vi "get data definition.vi"(10 "channel classification":T1, 11 "AppStateMachine runtime in":refnum<class "AppStateMachine runtime.lvclass">) -> (1 "valid?":bool, 2 "index cluster":variant, 3 "AppStateMachine runtime out":refnum<class "AppStateMachine runtime.lvclass">)   [LabVIEW 2017, in "AppStateMachine runtime.lvclass"]
uses:
  AppStateMachine runtime.lvclass
  <vilib>/NI/Tag Bus Module Framework/channel/channel classification.ctl
  input user data.ctl
  output user data.ctl
  parameter user data.ctl
  result user data.ctl
  <vilib>/NI/Tag Bus Module Framework/channel/TBM channel.lvclass
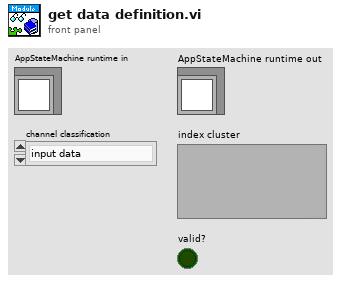
[diagram p1: front panel]
types:
  T1 = typedef "TBM channel.lvclass/channel classification.ctl" = enum16{"input data", "output data", "processing parameter", "processing result"}
  T2 = typedef "AppStateMachine runtime.lvclass/input user data.ctl" = cluster{"fmwk_placeholder":i32}
  T3 = typedef "AppStateMachine runtime.lvclass/output user data.ctl" = cluster{"fmwk_placeholder":i32}
  T4 = typedef "AppStateMachine runtime.lvclass/parameter user data.ctl" = cluster{"CPU":dbl, "Memory":dbl, "Disk":dbl}
  T5 = typedef "AppStateMachine runtime.lvclass/result user data.ctl" = cluster{"State":u16, "LED_Enable":bool, "LED_BlinksPerCycle":i32, "LED_GreenOrYellow":bool}
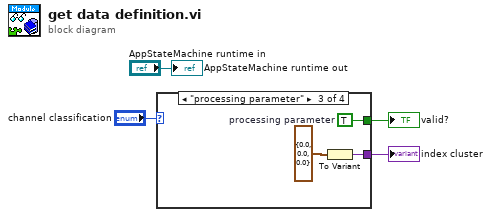
[diagram p0: block diagram]
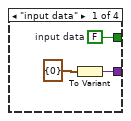
[diagram p2: hidden frame]
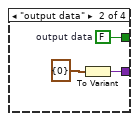
[diagram p3: hidden frame]
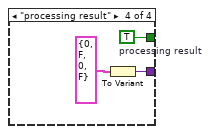
[diagram p4: hidden frame]
diagram:
  n1 = case shown="\"processing parameter\"" "channel classification" {
    tunnel: [w6 w10 w13 w16] -> w2
    tunnel: [w5 w9 w12 w15] -> w1
    frame "input data" {
      w5 = FALSE  # input data
      n2 = To Variant(anything=T2 {"fmwk_placeholder"=0} ("Inputs from system")) -> (Variant=w6:variant)
    }
    frame "output data" {
      w9 = FALSE  # output data
      n3 = To Variant(anything=T3 {"fmwk_placeholder"=0} ("Outputs to system")) -> (Variant=w10:variant)
    }
    frame "processing parameter" {
      w12 = TRUE  # processing parameter
      n4 = To Variant(anything=T4 {"CPU"=0.0, "Memory"=0.0, "Disk"=0.0} ("Parameters to process")) -> (Variant=w13:variant)
    }
    frame "processing result" {
      w15 = TRUE  # processing result
      n5 = To Variant(anything=T5 {"State"=0, "LED_Enable"=FALSE, "LED_BlinksPerCycle"=0, "LED_GreenOrYellow"=FALSE} ("Results from processing")) -> (Variant=w16:variant)
    }
  }
  "index cluster" <- w2
  "valid?" <- w1
  "AppStateMachine runtime out" <- "AppStateMachine runtime in"
